vi "3_1_Approx. of a real signal in terms of another real signal.vi"() -> ()   [LabVIEW 2009]
uses:
  <vilib>/Analysis/NI_AALBase.lvlib
panel:
  out "Area =":dbl=63.641031907547855 format="%#.5f"
  in  "Ring":u16(ring) items=["Approximation: C.f2(t)", "Area under the curve f1(t).f2(t)"]
  out "Power in the interval":dbl=15.915494309189533
  out "Power in the interval":dbl=7.957747154594758
  out "Error e":dbl=3.023367961652013
  in  "T2":enum16{"0", "pi/2", "pi", "3pi/2", "2pi"}(ring)=enum."2pi"
  in  "T1":enum16{"0", "-pi/2", "-pi", "-3pi/2", "-2pi"}(ring)
  in  "Frequency":dbl=1.0 min=-49.0 max=49.0
  in  "Frequency":dbl=1.0 min=-49.0 max=49.0
  in  "stop":bool
  in  "Signal 2: f2(t)":T1(ring)=enum."SINE"
  in  "Signal 1: f1(t)":T2(ring)
  out "C":dbl=1.2728206381509586 format="%#.5f"
  out "Approximation: f1(t) ~ C.f2(t) {The yellow curve}":cluster{"phase":dbl, dbl, dbl[][]}(graph)={"phase"=0.0, 3.6, [[0.0, 0.07992106913713087, 0.1595267263268409, 0.23850280440856755, 0.31653762088286036, 0.39332320797981174, 0.468556528067148, 0.5419406696013188, 0.6131860189017142, 0.6820114031235494, 0.748145199918628, 0.8113264094046575, 0.8713056842125456, 0.9278463135465496, 0.9807251573736447, 1.0297335270552912, 1.07467800894615, 1.1153812277093784, 1.1516825463360498, 1.18343870010604, 1.210524361988425, 1.232832637250017, 1.2502754853200402, 1.2627840672460413, 1.270309017369786, 1.2728206381509586, 1.270309017369786, 1.2627840672460413, 1.2502754853200404, 1.2328326372500171, 1.2105243619884254, 1.1834387001060405, 1.1516825463360505, 1.115381227709379, 1.0746780089461507, 1.0297335270552923, 0.9807251573736459, 0.9278463135465508, 0.8713056842125472, 0.8113264094046592, 0.7481451999186299, 0.6820114031235517, 0.6131860189017166, 0.5419406696013215, 0.4685565280671508, 0.39332320797981485, 0.3165376208828636, 0.23850280440857097, 0.15952672632684445, 0.0799210691371346, 3.855912752818189e-15, -0.0799210691371269, -0.1595267263268368, -0.2385028044085634, -0.31653762088285614, -0.39332320797980747, -0.4685565280671437, -0.5419406696013145, -0.6131860189017099, -0.6820114031235451, -0.7481451999186237, -0.8113264094046533, -0.8713056842125415, -0.9278463135465456, -0.9807251573736409, -1.0297335270552876, -1.0746780089461467, -1.1153812277093753, -1.1516825463360472, -1.1834387001060376, -1.210524361988423, -1.2328326372500154, -1.250275485320039, -1.2627840672460406, -1.2703090173697857, -1.2728206381509586, -1.2703090173697864, -1.2627840672460418, -1.2502754853200408, -1.2328326372500178, -1.2105243619884256, -1.1834387001060407, -1.1516825463360505, -1.1153812277093789, -1.07467800894615, -1.029733527055291, -0.9807251573736443, -0.9278463135465487, -0.8713056842125443, -0.8113264094046558, -0.7481451999186258, -0.6820114031235468, -0.6131860189017112, -0.5419406696013153, -0.4685565280671439, -0.3933232079798071, -0.3165376208828551, -0.23850280440856172, -0.15952672632683448, -0.07992106913712395], [1.0, 1.0, 1.0, 1.0, 1.0, 1.0, 1.0, 1.0, 1.0, 1.0, 1.0, 1.0, 1.0, 1.0, 1.0, 1.0, 1.0, 1.0, 1.0, 1.0, 1.0, 1.0, 1.0, 1.0, 1.0, 1.0, 1.0, 1.0, 1.0, 1.0, 1.0, 1.0, 1.0, 1.0, 1.0, 1.0, 1.0, 1.0, 1.0, 1.0, 1.0, 1.0, 1.0, 1.0, 1.0, 1.0, 1.0, 1.0, 1.0, 1.0, 1.0, -1.0, -1.0, -1.0, -1.0, -1.0, -1.0, -1.0, -1.0, -1.0, -1.0, -1.0, -1.0, -1.0, -1.0, -1.0, -1.0, -1.0, -1.0, -1.0, -1.0, -1.0, -1.0, -1.0, -1.0, -1.0, -1.0, -1.0, -1.0, -1.0, -1.0, -1.0, -1.0, -1.0, -1.0, -1.0, -1.0, -1.0, -1.0, -1.0, -1.0, -1.0, -1.0, -1.0, -1.0, -1.0, -1.0, -1.0, -1.0, -1.0], [0.0, 0.06279051952931337, 0.12533323356430426, 0.18738131458572463, 0.2486898871648548, 0.3090169943749474, 0.368124552684678, 0.42577929156507266, 0.4817536741017153, 0.5358267949789967, 0.5877852522924732, 0.6374239897486899, 0.6845471059286888, 0.7289686274214117, 0.7705132427757894, 0.8090169943749476, 0.8443279255020152, 0.8763066800438637, 0.9048270524660196, 0.9297764858882515, 0.9510565162951535, 0.9685831611286311, 0.9822872507286886, 0.9921147013144778, 0.9980267284282716, 1.0, 0.9980267284282716, 0.9921147013144779, 0.9822872507286888, 0.9685831611286313, 0.9510565162951539, 0.9297764858882518, 0.90482705246602, 0.8763066800438643, 0.8443279255020159, 0.8090169943749483, 0.7705132427757903, 0.7289686274214127, 0.6845471059286901, 0.6374239897486912, 0.5877852522924748, 0.5358267949789984, 0.4817536741017172, 0.42577929156507477, 0.3681245526846802, 0.30901699437494984, 0.24868988716485732, 0.18738131458572732, 0.12533323356430706, 0.0627905195293163, 3.0294235002503722e-15, -0.06279051952931025, -0.12533323356430104, -0.18738131458572135, -0.24868988716485146, -0.30901699437494407, -0.3681245526846746, -0.4257792915650693, -0.48175367410171194, -0.5358267949789933, -0.5877852522924699, -0.6374239897486865, -0.6845471059286856, -0.7289686274214086, -0.7705132427757864, -0.8090169943749448, -0.8443279255020126, -0.8763066800438613, -0.9048270524660175, -0.9297764858882496, -0.951056516295152, -0.9685831611286299, -0.9822872507286877, -0.9921147013144772, -0.9980267284282713, -1.0, -0.9980267284282718, -0.9921147013144782, -0.9822872507286892, -0.9685831611286317, -0.9510565162951542, -0.929776485888252, -0.90482705246602, -0.876306680043864, -0.8443279255020153, -0.8090169943749475, -0.770513242775789, -0.728968627421411, -0.6845471059286878, -0.6374239897486885, -0.5877852522924716, -0.5358267949789947, -0.48175367410171294, -0.4257792915650699, -0.36812455268467476, -0.30901699437494373, -0.24868988716485066, -0.18738131458572005, -0.12533323356429923, -0.06279051952930793]]}
  out "Signal 2: f2(t)":cluster{"phase":dbl, dbl, "sawtooth wave":dbl[]}(graph)={"phase"=0.0, 3.6, "sawtooth wave"=[0.0, 0.06279051952931337, 0.12533323356430426, 0.18738131458572463, 0.2486898871648548, 0.3090169943749474, 0.368124552684678, 0.42577929156507266, 0.4817536741017153, 0.5358267949789967, 0.5877852522924732, 0.6374239897486899, 0.6845471059286888, 0.7289686274214117, 0.7705132427757894, 0.8090169943749476, 0.8443279255020152, 0.8763066800438637, 0.9048270524660196, 0.9297764858882515, 0.9510565162951535, 0.9685831611286311, 0.9822872507286886, 0.9921147013144778, 0.9980267284282716, 1.0, 0.9980267284282716, 0.9921147013144779, 0.9822872507286888, 0.9685831611286313, 0.9510565162951539, 0.9297764858882518, 0.90482705246602, 0.8763066800438643, 0.8443279255020159, 0.8090169943749483, 0.7705132427757903, 0.7289686274214127, 0.6845471059286901, 0.6374239897486912, 0.5877852522924748, 0.5358267949789984, 0.4817536741017172, 0.42577929156507477, 0.3681245526846802, 0.30901699437494984, 0.24868988716485732, 0.18738131458572732, 0.12533323356430706, 0.0627905195293163, 3.0294235002503722e-15, -0.06279051952931025, -0.12533323356430104, -0.18738131458572135, -0.24868988716485146, -0.30901699437494407, -0.3681245526846746, -0.4257792915650693, -0.48175367410171194, -0.5358267949789933, -0.5877852522924699, -0.6374239897486865, -0.6845471059286856, -0.7289686274214086, -0.7705132427757864, -0.8090169943749448, -0.8443279255020126, -0.8763066800438613, -0.9048270524660175, -0.9297764858882496, -0.951056516295152, -0.9685831611286299, -0.9822872507286877, -0.9921147013144772, -0.9980267284282713, -1.0, -0.9980267284282718, -0.9921147013144782, -0.9822872507286892, -0.9685831611286317, -0.9510565162951542, -0.929776485888252, -0.90482705246602, -0.876306680043864, -0.8443279255020153, -0.8090169943749475, -0.770513242775789, -0.728968627421411, -0.6845471059286878, -0.6374239897486885, -0.5877852522924716, -0.5358267949789947, -0.48175367410171294, -0.4257792915650699, -0.36812455268467476, -0.30901699437494373, -0.24868988716485066, -0.18738131458572005, -0.12533323356429923, -0.06279051952930793]}
  out "Signal 1: f1(t)":cluster{"phase":dbl, dbl, "triangle wave":dbl[]}(graph)={"phase"=0.0, 3.6, "triangle wave"=[1.0, 1.0, 1.0, 1.0, 1.0, 1.0, 1.0, 1.0, 1.0, 1.0, 1.0, 1.0, 1.0, 1.0, 1.0, 1.0, 1.0, 1.0, 1.0, 1.0, 1.0, 1.0, 1.0, 1.0, 1.0, 1.0, 1.0, 1.0, 1.0, 1.0, 1.0, 1.0, 1.0, 1.0, 1.0, 1.0, 1.0, 1.0, 1.0, 1.0, 1.0, 1.0, 1.0, 1.0, 1.0, 1.0, 1.0, 1.0, 1.0, 1.0, 1.0, -1.0, -1.0, -1.0, -1.0, -1.0, -1.0, -1.0, -1.0, -1.0, -1.0, -1.0, -1.0, -1.0, -1.0, -1.0, -1.0, -1.0, -1.0, -1.0, -1.0, -1.0, -1.0, -1.0, -1.0, -1.0, -1.0, -1.0, -1.0, -1.0, -1.0, -1.0, -1.0, -1.0, -1.0, -1.0, -1.0, -1.0, -1.0, -1.0, -1.0, -1.0, -1.0, -1.0, -1.0, -1.0, -1.0, -1.0, -1.0, -1.0]}
  out "Area under the curve f1(t).f2(t)":cluster{"phase":dbl, dbl, dbl[]}(graph)={"phase"=0.0, 3.6, [0.0, 0.06279051952931337, 0.12533323356430426, 0.18738131458572463, 0.2486898871648548, 0.3090169943749474, 0.368124552684678, 0.42577929156507266, 0.4817536741017153, 0.5358267949789967, 0.5877852522924732, 0.6374239897486899, 0.6845471059286888, 0.7289686274214117, 0.7705132427757894, 0.8090169943749476, 0.8443279255020152, 0.8763066800438637, 0.9048270524660196, 0.9297764858882515, 0.9510565162951535, 0.9685831611286311, 0.9822872507286886, 0.9921147013144778, 0.9980267284282716, 1.0, 0.9980267284282716, 0.9921147013144779, 0.9822872507286888, 0.9685831611286313, 0.9510565162951539, 0.9297764858882518, 0.90482705246602, 0.8763066800438643, 0.8443279255020159, 0.8090169943749483, 0.7705132427757903, 0.7289686274214127, 0.6845471059286901, 0.6374239897486912, 0.5877852522924748, 0.5358267949789984, 0.4817536741017172, 0.42577929156507477, 0.3681245526846802, 0.30901699437494984, 0.24868988716485732, 0.18738131458572732, 0.12533323356430706, 0.0627905195293163, 3.0294235002503722e-15, 0.06279051952931025, 0.12533323356430104, 0.18738131458572135, 0.24868988716485146, 0.30901699437494407, 0.3681245526846746, 0.4257792915650693, 0.48175367410171194, 0.5358267949789933, 0.5877852522924699, 0.6374239897486865, 0.6845471059286856, 0.7289686274214086, 0.7705132427757864, 0.8090169943749448, 0.8443279255020126, 0.8763066800438613, 0.9048270524660175, 0.9297764858882496, 0.951056516295152, 0.9685831611286299, 0.9822872507286877, 0.9921147013144772, 0.9980267284282713, 1.0, 0.9980267284282718, 0.9921147013144782, 0.9822872507286892, 0.9685831611286317, 0.9510565162951542, 0.929776485888252, 0.90482705246602, 0.876306680043864, 0.8443279255020153, 0.8090169943749475, 0.770513242775789, 0.728968627421411, 0.6845471059286878, 0.6374239897486885, 0.5877852522924716, 0.5358267949789947, 0.48175367410171294, 0.4257792915650699, 0.36812455268467476, 0.30901699437494373, 0.24868988716485066, 0.18738131458572005, 0.12533323356429923, 0.06279051952930793]}
  out "ST":string
  # "Program Developed by Indranil Sinharoy"
  # "APPROXIMATION OF ONE REAL SIGNAL IN TERMS OF ANOTHER REAL SIGNAL IN ONE DIMENSION"
  # "The real signal f1(t) is approxiamted in terms of another real signal f2(t) over an interval [T1,T2] :"
  # "The signal f1(t) is approximated in terms of f2(t) over a certain interval ( T1 < t <T2 ) as follows :\n\n                          f1(t) ~ C . f2(t)          for   (T1 <  t < T2)\n \nThat is we say that f1(t) has a component of waveform f2(t), and this component (C.f2) has a \nmagnitude C. If C vanishes, then the signal f1(t) contains no component of signal f2(t) and we \nsay that the two functions are orthogonal over the interval (T1,T2)."
  # "Interval:"
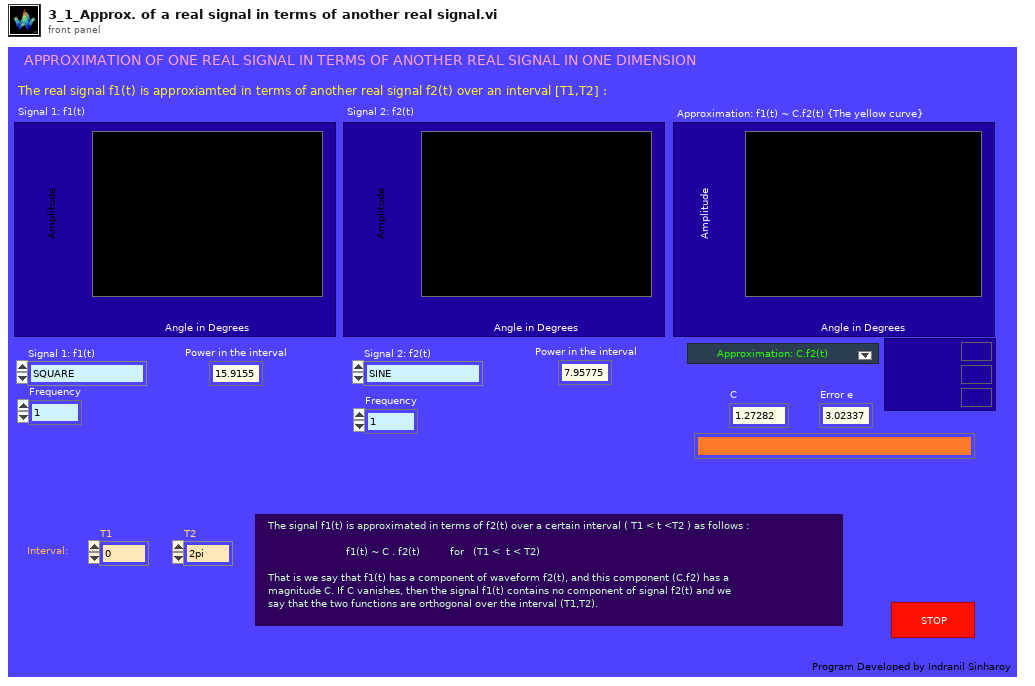
[diagram p1: front panel]
types:
  T1 = enum16{"SQUARE", "SINE", "COS", "TRIANGULAR", "RAMP", "SAWTOOTH", "NULL SIGNAL"}
  T2 = enum16{"SQUARE", "COS", "SINE", "SAWTOOTH", "RAMP", "TRIANGULAR"}
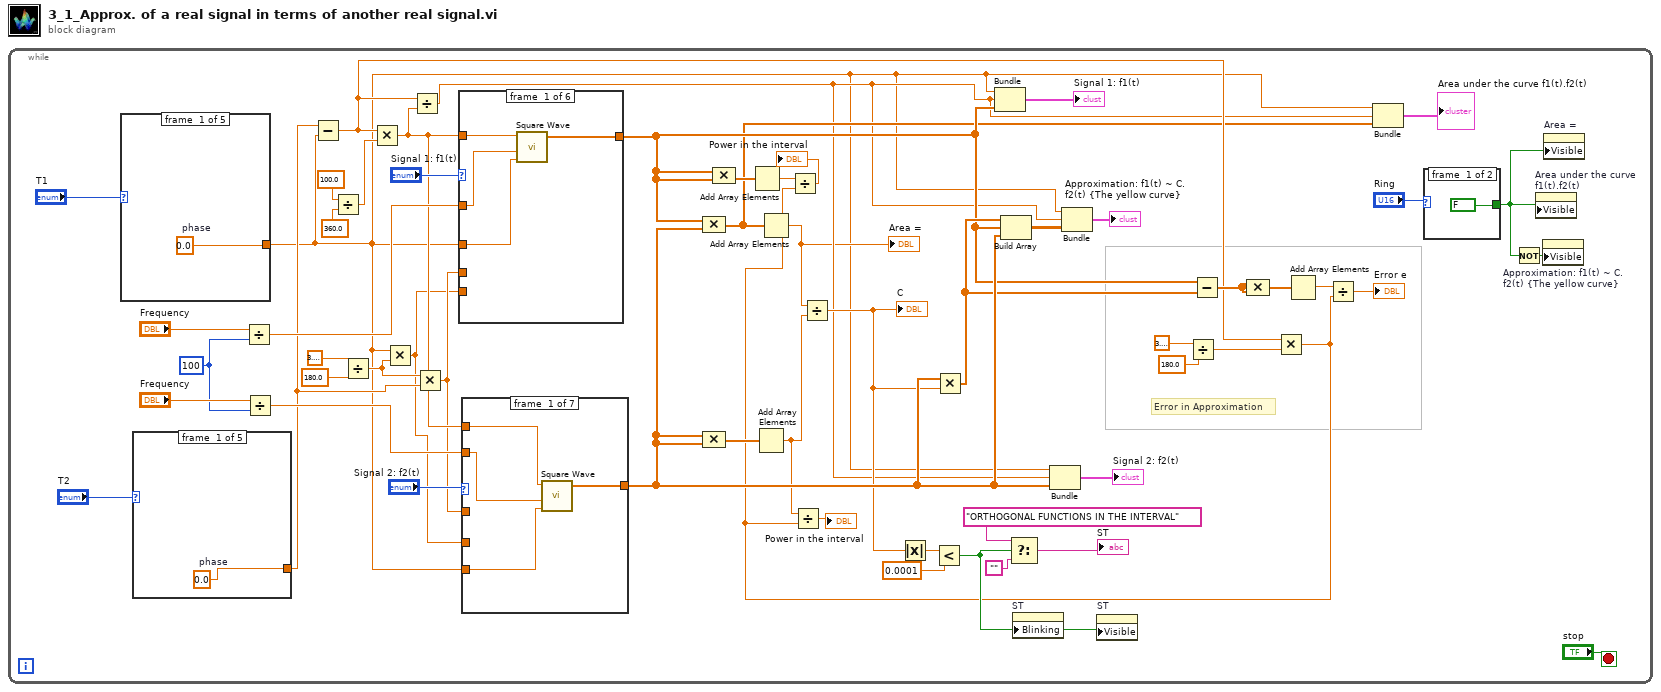
[diagram p0: block diagram]
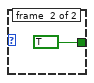
[diagram p2: hidden frame]
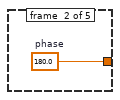
[diagram p3: hidden frame]
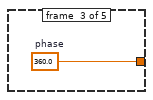
[diagram p4: hidden frame]
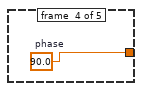
[diagram p5: hidden frame]
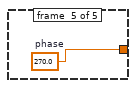
[diagram p6: hidden frame]
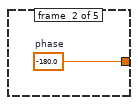
[diagram p7: hidden frame]
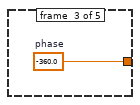
[diagram p8: hidden frame]
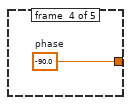
[diagram p9: hidden frame]
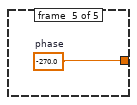
[diagram p10: hidden frame]
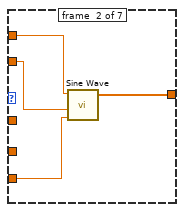
[diagram p11: hidden frame]
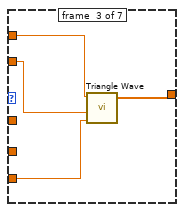
[diagram p12: hidden frame]
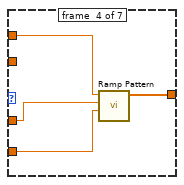
[diagram p13: hidden frame]
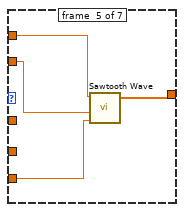
[diagram p14: hidden frame]
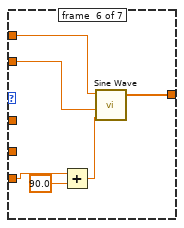
[diagram p15: hidden frame]
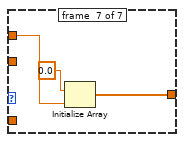
[diagram p16: hidden frame]
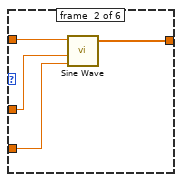
[diagram p17: hidden frame]
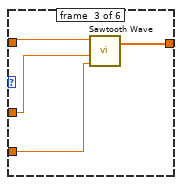
[diagram p18: hidden frame]
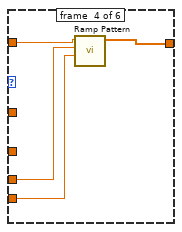
[diagram p19: hidden frame]
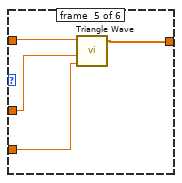
[diagram p20: hidden frame]
diagram:
  n1 = while {
    stop <- "stop" stop-if-true
    w47 = 100
    # "Error in Approximation"
    n2 = case shown="\"-pi\"" "T1" {
      tunnel: [w65 w66 w67 w68 w69] -> w3
      frame #0 {
        w65 = 0.0  # phase
      }
      frame #1 {
        w66 = -180.0  # phase
      }
      frame #2 {
        w67 = -360.0  # phase
      }
      frame #3 {
        w68 = -90.0  # phase
      }
      frame #4 {
        w69 = -270.0  # phase
      }
    }
    n3 = case shown="\"2pi\"" "T2" {
      tunnel: [w60 w61 w62 w63 w64] -> w4
      frame #0 {
        w60 = 0.0  # phase
      }
      frame #1 {
        w61 = 180.0  # phase
      }
      frame #2 {
        w62 = 360.0  # phase
      }
      frame #3 {
        w63 = 90.0  # phase
      }
      frame #4 {
        w64 = 270.0  # phase
      }
    }
    n4 = Divide(x="Frequency", y=w47) -> (x/y=w45:dbl)
    n5 = Divide(x="Frequency", y=w47) -> (x/y=w49:dbl)
    n6 = Subtract(x=w4, y=w3) -> (x-y=w18:dbl)
    n7 = Divide(x=100.0, y=360.0) -> (x/y=w44:dbl)
    n8 = Divide(x=3.141592653589793, y=180.0) -> (x/y=w5:dbl)
    n9 = Multiply(x=w18, y=w44) -> (x*y=w42:dbl)
    n10 = Multiply(x=w3, y=w5) -> (x*y=w1:dbl)
    n11 = Divide(x=w18, y=w42) -> (x/y=w13:dbl)
    n12 = Multiply(x=w5, y=w4) -> (x*y=w2:dbl)
    n13 = case shown="\"RAMP\"" "Signal 1: f1(t)" {
      tunnel: [w102 w106 w110 w114 w118 w123] -> w22
      tunnel: w3 -> [w101 w105 w109 _ w117 w121]
      tunnel: w42 -> [w100 w104 w108 w113 w116 w124]
      tunnel: w45 -> [w99 w103 w107 _ w115 w122]
      tunnel: w1 -> [_ _ _ w112 _ _]
      tunnel: w2 -> [_ _ _ w111 _ _]
      frame #0 {
        n14 = call <vilib>:"Square Wave.vi"("samples"=w100, "frequency"=w99, "phase in"=w101) -> ("square wave"=w102:dbl[])  [unwired: 3 in, 2 out]
      }
      frame #1 {
        n15 = call <vilib>:"Sine Wave.vi"("samples"=w104, "frequency"=w103, "phase in"=w105) -> ("sine wave"=w106:dbl[])  [unwired: 2 in, 2 out]
      }
      frame #2 {
        n16 = call <vilib>:"Sawtooth Wave.vi"("samples"=w108, "frequency"=w107, "phase in"=w109) -> ("sawtooth wave"=w110:dbl[])  [unwired: 2 in, 2 out]
      }
      frame #3 {
        n17 = call <vilib>:"Ramp Pattern.vi"("start"=w112, "end"=w111, "samples"=w113) -> ("Ramp Pattern"=w114:dbl[])  [unwired: 7 in, 1 out]
      }
      frame #4 {
        n18 = call <vilib>:"Triangle Wave.vi"("samples"=w116, "frequency"=w115, "phase in"=w117) -> ("triangle wave"=w118:dbl[])  [unwired: 2 in, 2 out]
      }
      frame #5 {
        n19 = Add(x=w121, y=90.0) -> (x+y=w120:dbl)
        n20 = call <vilib>:"Sine Wave.vi"("samples"=w124, "frequency"=w122, "phase in"=w120) -> ("sine wave"=w123:dbl[])  [unwired: 2 in, 2 out]
      }
    }
    n21 = case shown="\"RAMP\"" "Signal 2: f2(t)" {
      tunnel: [w73 w77 w81 w85 w89 w90 w96] -> w41
      tunnel: w3 -> [w72 w76 w80 _ w88 w91 _]
      tunnel: w42 -> [w71 w75 w79 w84 w87 w92 w98]
      tunnel: w49 -> [w70 w74 w78 _ w86 w93 _]
      tunnel: w2 -> [_ _ _ w83 _ _ _]
      tunnel: w1 -> [_ _ _ w82 _ _ _]
      frame #0 {
        n22 = call <vilib>:"Square Wave.vi"("samples"=w71, "frequency"=w70, "phase in"=w72) -> ("square wave"=w73:dbl[])  [unwired: 3 in, 2 out]
      }
      frame #1 {
        n23 = call <vilib>:"Sine Wave.vi"("samples"=w75, "frequency"=w74, "phase in"=w76) -> ("sine wave"=w77:dbl[])  [unwired: 2 in, 2 out]
      }
      frame #2 {
        n24 = call <vilib>:"Triangle Wave.vi"("samples"=w79, "frequency"=w78, "phase in"=w80) -> ("triangle wave"=w81:dbl[])  [unwired: 2 in, 2 out]
      }
      frame #3 {
        n25 = call <vilib>:"Ramp Pattern.vi"("start"=w82, "end"=w83, "samples"=w84) -> ("Ramp Pattern"=w85:dbl[])  [unwired: 7 in, 1 out]
      }
      frame #4 {
        n26 = call <vilib>:"Sawtooth Wave.vi"("samples"=w87, "frequency"=w86, "phase in"=w88) -> ("sawtooth wave"=w89:dbl[])  [unwired: 2 in, 2 out]
      }
      frame #5 {
        n27 = Add(x=w91, y=90.0) -> (x+y=w94:dbl)
        n28 = call <vilib>:"Sine Wave.vi"("samples"=w92, "frequency"=w93, "phase in"=w94) -> ("sine wave"=w90:dbl[])  [unwired: 2 in, 2 out]
      }
      frame #6 {
        n29 = Initialize Array(0.0 ("element"), w98) -> (w96:dbl[])
      }
    }
    n30 = Compound Arithmetic op=MULTIPLY(w22, w41) -> (w14:dbl[])
    n31 = Compound Arithmetic op=MULTIPLY(w41, w41) -> (w57:dbl[])
    n32 = Compound Arithmetic op=MULTIPLY(w22, w22) -> (w21:dbl[])
    n33 = Add Array Elements(numeric array=w21) -> (sum=w16:dbl)
    n34 = Add Array Elements(numeric array=w57) -> (sum=w20:dbl)
    n35 = Add Array Elements(numeric array=w14) -> (sum=w9:dbl)
    "Area =" <- w9
    n36 = Divide(x=w9, y=w20) -> (x/y=w34:dbl)
    "C" <- w34
    n37 = Absolute Value(x=w34) -> (abs(x)=w33:dbl)
    n38 = Less?(x=w33, y=0.0001) -> (x < y?=w31:bool)
    n39 = Multiply(x=w41, y=w34) -> (x*y=w30:dbl[])
    n40 = Bundle("phase"=w3, w13, "sine wave"=w22) -> (→"Signal 1: f1(t)":cluster{"phase":dbl, dbl, "sine wave":dbl[]})  [unwired: 1 in]
    n41 = Build Array(w30, w22, w41) -> (w39:dbl[][])
    n42 = Select(t="ORTHOGONAL FUNCTIONS IN THE INTERVAL", s=w31, f="") -> (s? t:f=→"ST":string)
    n43 = property on="ST" class="Str"("Blinking"=w31) -> ()  [unwired: 2 in, 2 out]
    n44 = Bundle("phase"=w3, w13, "sine wave"=w41) -> (→"Signal 2: f2(t)":cluster{"phase":dbl, dbl, "sine wave":dbl[]})  [unwired: 1 in]
    n45 = Bundle("phase"=w3, w13, w39) -> (→"Approximation: f1(t) ~ C.f2(t) {The yellow curve}":cluster{"phase":dbl, dbl, dbl[][]})  [unwired: 1 in]
    n46 = property on="ST" class="Str"("Visible"=w31) -> ()  [unwired: 2 in, 2 out]
    n47 = Divide(x=3.141592653589793, y=180.0) -> (x/y=w26:dbl)
    n48 = Subtract(x=w22, y=w30) -> (x-y=w29:dbl[])
    n49 = Compound Arithmetic op=MULTIPLY(w29, w29) -> (w28:dbl[])
    n50 = Multiply(x=w18, y=w26) -> (x*y=w15:dbl)
    n51 = Divide(x=w16, y=w15) -> (x/y=→"Power in the interval":dbl)
    n52 = Divide(x=w20, y=w15) -> (x/y=→"Power in the interval":dbl)
    n53 = Add Array Elements(numeric array=w28) -> (sum=w27:dbl)
    n54 = Divide(x=w27, y=w15) -> (x/y=→"Error e":dbl)
    n55 = Bundle("phase"=w3, w13, w14) -> (→"Area under the curve f1(t).f2(t)":cluster{"phase":dbl, dbl, dbl[]})  [unwired: 1 in]
    n56 = case shown="0, Default" "Ring" {
      tunnel: [FALSE TRUE] -> w8
      frame #0 {
      }
      frame #1 {
      }
    }
    n57 = Not(x=w8) -> (.not. x?=w10:bool)
    n58 = property on="Area under the curve f1(t).f2(t)" class="WFGraph (strict)"("Visible"=w8) -> ()  [unwired: 2 in, 2 out]
    n59 = property on="Approximation: f1(t) ~ C.f2(t) {The yellow curve}" class="WFGraph (strict)"("Visible"=w10) -> ()  [unwired: 2 in, 2 out]
    n60 = property on="Area =" class="DigNum (strict)"("Visible"=w8) -> ()  [unwired: 2 in, 2 out]
  }
